vi "GetPhdwf.vi"(0 "object in":refnum<class "AD2_SDK.lvclass">, 5 "error in (no error)":errorcluster) -> (14 "object out":refnum<class "AD2_SDK.lvclass">, 15 "phdwf":i32=1, 19 "error out":errorcluster)   [LabVIEW 2019, in "AD2_SDK.lvclass"]
uses:
  AD2_SDK.lvclass
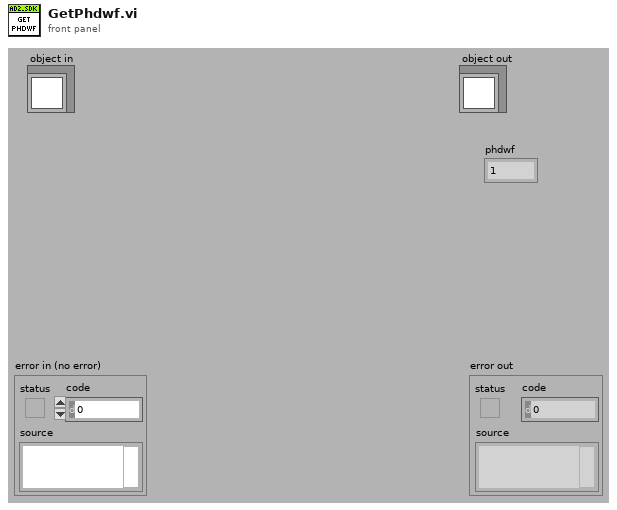
[diagram p1: front panel]
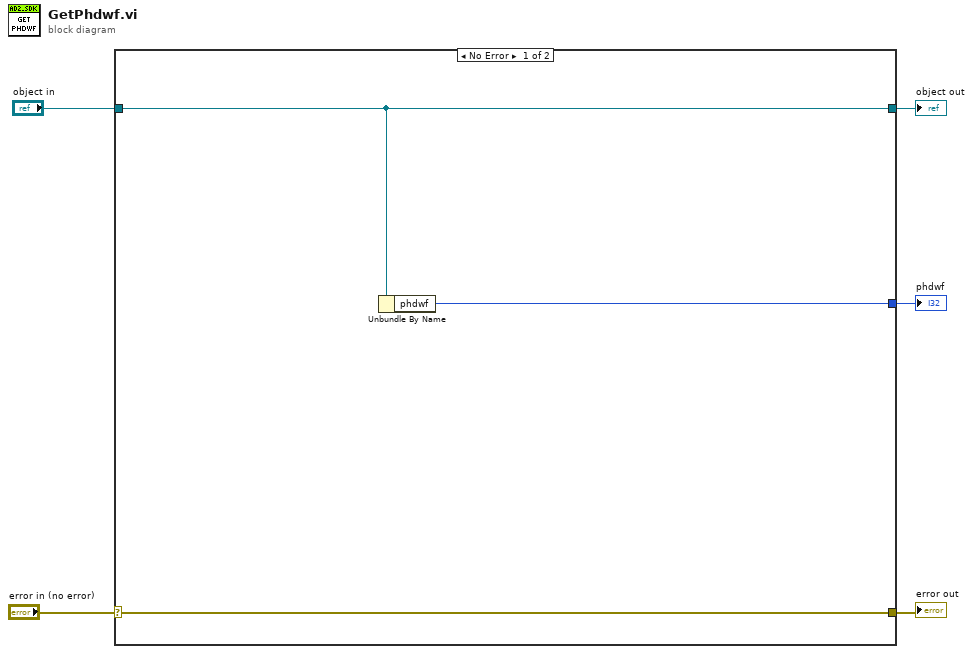
[diagram p0: block diagram]
diagram:
  n1 = case shown="No Error" "error in (no error)" {
    selector: "error in (no error)" -> [w7 w10]
    tunnel: [w7 w10] -> w4
    tunnel: [w6 w9] -> w2
    tunnel: "object in" -> [w6 w9]
    tunnel: [w8 _] -> w1
    frame No Error {
      n2 = Unbundle By Name(w6) -> ("phdwf"=w8:i32)
    }
    frame Error {
    }
  }
  "error out" <- w4
  "object out" <- w2
  "phdwf" <- w1
